vi "ReplaceAngles.vi"(9 "Angle2In":dbl, 10 "Angle1In":dbl, 11 "Comm":T1={"url"="https://rogers.onshape.com/api/partstudios/d/78f5bf641b1754cc5a2885a6/w/2816a0ac3f158e698c5324a2/e/990ec2d1208dce12e8c8d73d/sketches?", "sent headers"="Accept: application/json\r\nAuthorization: On 5WRzTWmAmwc94xTxHfKZAg5i:HmacSHA256:lDyQC1x2JlGNCtdzVGE5L8N41PUpGQIlxBBiesg5jjs=\r\nContent-Type: application/json\r\nDate: Thu, 16 Apr 2020 23:19:12 GMT\r\nOn-Nonce: nlS7Y9rr4jS35A8DK9B3OToU\r\nUser_agent: Onshape Python Sample App", "sent body"="", "headers"="HTTP/1.1 200 OK\r\nServer: nginx\r\nDate: Thu, 16 Apr 2020 23:19:12 GMT\r\nContent-Type: application/json;charset=UTF-8;qs=0.9\r\nContent-Length: 2372\r\nConnection: keep-alive\r\nVary: Accept-Encoding\r\nOn-Version: 1.111.25149.0c1f2eb083aa\r\nOn-Request-Id: a78cc699fde7b461387b36e3\r\nDeprecation: version=UNDEFINED, message=\"You specified mediatype application/json;charset=UTF-8;qs=0.9 and this endpoint will currently accept application/vnd.onshape.v1+json;charset=UTF-8;qs=0.1. Please consider updating to the latest version by specifying application/vnd.onshape.v1+json;charset=UTF-8;qs=0.1 within the Accept header.\r\nSet-Cookie: _u=webservice-3e25a82e; Path=/; Secure; HttpOnly;\r\nX-Frame-Options: SAMEORIGIN\r\nStrict-Transport-Security: max-age=31536000; includeSubDomains\r\nX-Content-Type-Options: nosniff\r\nX-XSS-Protection: 1; mode=block\r\nContent-Security-Policy-Report-Only: object-src 'self' https://embedwistia-a.akamaihd.net; report-uri /api/csp\r\n\r\n", "body"="{\n  \"sketches\" : [ {\n    \"sketch\" : \"Sketch 1\",\n    \"featureId\" : \"FbqM6rYzUBbMRp8_0\",\n    \"transformMatrix\" : [ 1.0, 0.0, 0.0, 0.0, 0.0, 1.0, 0.0, 0.0, 0.0, 0.0, 1.0, 0.0, 0.0, 0.0, 0.0, 1.0 ],\n    \"featuresUsed\" : [ ],\n    \"geomEntities\" : [ {\n      \"id\" : \"C471k0qsEi0Q.start\",\n      \"entityType\" : \"point\",\n      \"point\" : [ 0.017283352091908455, -0.007151731755584478 ]\n    }, {\n      \"id\" : \"C471k0qsEi0Q.end\",\n      \"entityType\" : \"point\",\n      \"point\" : [ -0.04529430344700813, 0.05423396825790405 ]\n    }, {\n      \"id\" : \"C471k0qsEi0Q.0.internal\",\n      \"entityType\" : \"point\",\n      \"point\" : [ 0.017283352091908455, -0.007151731755584478 ]\n    }, {\n      \"id\" : \"C471k0qsEi0Q.1.internal\",\n      \"entityType\" : \"point\",\n      \"point\" : [ 0.05095608904957771, 0.022945139557123184 ]\n    }, {\n      \"id\" : \"C471k0qsEi0Q.2.internal\",\n      \"entityType\" : \"point\",\n      \"point\" : [ 0.02443508431315422, 0.05780983343720436 ]\n    }, {\n      \"id\" : \"C471k0qsEi0Q.3.internal\",\n      \"entityType\" : \"point\",\n      \"point\" : [ -0.018177319318056107, 0.039334528148174286 ]\n    }, {\n      \"id\" : \"C471k0qsEi0Q.4.internal\",\n      \"entityType\" : \"point\",\n      \"point\" : [ -0.04529430344700813, 0.05423396825790405 ]\n    }, {\n      \"id\" : \"C471k0qsEi0Q.startDerivative\",\n      \"entityType\" : \"point\",\n      \"point\" : [ 0.03353424071398461, 8.902966705931049E-4 ],\n      \"isConstruction\" : true\n    }, {\n      \"id\" : \"C471k0qsEi0Q.endDerivative\",\n      \"entityType\" : \"point\",\n      \"point\" : [ -0.0368764138795279, 0.04584760236142172 ],\n      \"isConstruction\" : true\n    }, {\n      \"id\" : \"C471k0qsEi0Q\",\n      \"entityType\" : \"interpolatedSplineSegment\",\n      \"periodic\" : false,\n      \"startHandle\" : [ 0.03353424071398461, 8.902966705931043E-4 ],\n      \"endHandle\" : [ -0.03687641387952791, 0.045847602361421734 ],\n      \"startDerivative\" : [ 0.18655982097041743, 0.0923222980796617 ],\n      \"endDerivative\" : [ -0.1167534466674709, 0.11631622339302505 ],\n      \"interpolationPoints\" : [ [ 0.017283352091908455, -0.007151731755584478 ], [ 0.05095608904957771, 0.022945139557123184 ], [ 0.02443508431315422, 0.05780983343720436 ], [ -0.018177319318056107, 0.039334528148174286 ], [ -0.04529430344700813, 0.05423396825790405 ] ],\n      \"startParameter\" : 0.0,\n      \"endParameter\" : 1.0,\n      \"endPointIds\" : [ \"C471k0qsEi0Q.start\", \"C471k0qsEi0Q.end\" ]\n    } ]\n  } ]\n}", "Sent"="get https://rogers.onshape.com/api/partstudios/d/78f5bf641b1754cc5a2885a6/w/2816a0ac3f158e698c5324a2/e/990ec2d1208dce12e8c8d73d/sketches? \n\nAccept: application/json\r\nAuthorization: On 5WRzTWmAmwc94xTxHfKZAg5i:HmacSHA256:lDyQC1x2JlGNCtdzVGE5L8N41PUpGQIlxBBiesg5jjs=\r\nContent-Type: application/json\r\nDate: Thu, 16 Apr 2020 23:19:12 GMT\r\nOn-Nonce: nlS7Y9rr4jS35A8DK9B3OToU\r\nUser_agent: Onshape Python Sample App\n\n", "Received"="HTTP/1.1 200 OK\r\nServer: nginx\r\nDate: Thu, 16 Apr 2020 23:19:12 GMT\r\nContent-Type: application/json;charset=UTF-8;qs=0.9\r\nContent-Length: 2372\r\nConnection: keep-alive\r\nVary: Accept-Encoding\r\nOn-Version: 1.111.25149.0c1f2eb083aa\r\nOn-Request-Id: a78cc699fde7b461387b36e3\r\nDeprecation: version=UNDEFINED, message=\"You specified mediatype application/json;charset=UTF-8;qs=0.9 and this endpoint will currently accept application/vnd.onshape.v1+json;charset=UTF-8;qs=0.1. Please consider updating to the latest version by specifying application/vnd.onshape.v1+json;charset=UTF-8;qs=0.1 within the Accept header.\r\nSet-Cookie: _u=webservice-3e25a82e; Path=/; Secure; HttpOnly;\r\nX-Frame-Options: SAMEORIGIN\r\nStrict-Transport-Security: max-age=31536000; includeSubDomains\r\nX-Content-Type-Options: nosniff\r\nX-XSS-Protection: 1; mode=block\r\nContent-Security-Policy-Report-Only: object-src 'self' https://embedwistia-a.akamaihd.net; report-uri /api/csp\r\n\r\n\n\n{\n  \"sketches\" : [ {\n    \"sketch\" : \"Sketch 1\",\n    \"featureId\" : \"FbqM6rYzUBbMRp8_0\",\n    \"transformMatrix\" : [ 1.0, 0.0, 0.0, 0.0, 0.0, 1.0, 0.0, 0.0, 0.0, 0.0, 1.0, 0.0, 0.0, 0.0, 0.0, 1.0 ],\n    \"featuresUsed\" : [ ],\n    \"geomEntities\" : [ {\n      \"id\" : \"C471k0qsEi0Q.start\",\n      \"entityType\" : \"point\",\n      \"point\" : [ 0.017283352091908455, -0.007151731755584478 ]\n    }, {\n      \"id\" : \"C471k0qsEi0Q.end\",\n      \"entityType\" : \"point\",\n      \"point\" : [ -0.04529430344700813, 0.05423396825790405 ]\n    }, {\n      \"id\" : \"C471k0qsEi0Q.0.internal\",\n      \"entityType\" : \"point\",\n      \"point\" : [ 0.017283352091908455, -0.007151731755584478 ]\n    }, {\n      \"id\" : \"C471k0qsEi0Q.1.internal\",\n      \"entityType\" : \"point\",\n      \"point\" : [ 0.05095608904957771, 0.022945139557123184 ]\n    }, {\n      \"id\" : \"C471k0qsEi0Q.2.internal\",\n      \"entityType\" : \"point\",\n      \"point\" : [ 0.02443508431315422, 0.05780983343720436 ]\n    }, {\n      \"id\" : \"C471k0qsEi0Q.3.internal\",\n      \"entityType\" : \"point\",\n      \"point\" : [ -0.018177319318056107, 0.039334528148174286 ]\n    }, {\n      \"id\" : \"C471k0qsEi0Q.4.internal\",\n      \"entityType\" : \"point\",\n      \"point\" : [ -0.04529430344700813, 0.05423396825790405 ]\n    }, {\n      \"id\" : \"C471k0qsEi0Q.startDerivative\",\n      \"entityType\" : \"point\",\n      \"point\" : [ 0.03353424071398461, 8.902966705931049E-4 ],\n      \"isConstruction\" : true\n    }, {\n      \"id\" : \"C471k0qsEi0Q.endDerivative\",\n      \"entityType\" : \"point\",\n      \"point\" : [ -0.0368764138795279, 0.04584760236142172 ],\n      \"isConstruction\" : true\n    }, {\n      \"id\" : \"C471k0qsEi0Q\",\n      \"entityType\" : \"interpolatedSplineSegment\",\n      \"periodic\" : false,\n      \"startHandle\" : [ 0.03353424071398461, 8.902966705931043E-4 ],\n      \"endHandle\" : [ -0.03687641387952791, 0.045847602361421734 ],\n      \"startDerivative\" : [ 0.18655982097041743, 0.0923222980796617 ],\n      \"endDerivative\" : [ -0.1167534466674709, 0.11631622339302505 ],\n      \"interpolationPoints\" : [ [ 0.017283352091908455, -0.007151731755584478 ], [ 0.05095608904957771, 0.022945139557123184 ], [ 0.02443508431315422, 0.05780983343720436 ], [ -0.018177319318056107, 0.039334528148174286 ], [ -0.04529430344700813, 0.05423396825790405 ] ],\n      \"startParameter\" : 0.0,\n      \"endParameter\" : 1.0,\n      \"endPointIds\" : [ \"C471k0qsEi0Q.start\", \"C471k0qsEi0Q.end\" ]\n    } ]\n  } ]\n}"}) -> (3 "Payload":string="{\n  \"configurationParameters\" : [ {\n    \"type\" : 1826,\n    \"typeName\" : \"BTMConfigurationParameterQuantity\",\n    \"message\" : {\n      \"quantityType\" : \"ANGLE\",\n      \"rangeAndDefault\" : {\n        \"type\" : 181,\n        \"typeName\" : \"BTQuantityRange\",\n        \"message\" : {\n          \"units\" : \"degree\",\n          \"minValue\": 132.737430,\"maxValue\":132.737430,\"defaultValue\":132.737430,\"location\" : {\n            \"type\" : 226,\n            \"typeName\" : \"BTLocationInfo\",\n            \"message\" : {\n              \"document\" : \"\",\n              \"version\" : \"\",\n              \"topLevel\" : \"\",\n              \"parseNodeId\" : \"\",\n              \"character\" : 0,\n              \"line\" : 0,\n              \"column\" : 0,\n              \"endCharacter\" : 0,\n              \"endLine\" : 0,\n              \"endColumn\" : 0,\n              \"languageVersion\" : 0,\n              \"moduleIds\" : {\n                \"type\" : 1897,\n                \"typeName\" : \"BTDocumentVersionElementIds\",\n                \"message\" : {\n                  \"documentId\" : \"\",\n                  \"versionId\" : \"\",\n                  \"elementId\" : \"\"\n                }\n              },\n              \"elementMicroversion\" : \"\",\n              \"nodeId\" : \"+yByOudIvs1toQrG\"\n            }\n          }\n        }\n      },\n      \"parameterId\" : \"Angle1\",\n      \"parameterName\" : \"Angle1\",\n      \"hasUserCode\" : false,\n      \"nodeId\" : \"MLUebAszJBdGJ1Mml\"\n    }\n  }, {\n    \"type\" : 1826,\n    \"typeName\" : \"BTMConfigurationParameterQuantity\",\n    \"message\" : {\n      \"quantityType\" : \"ANGLE\",\n      \"rangeAndDefault\" : {\n        \"type\" : 181,\n        \"typeName\" : \"BTQuantityRange\",\n        \"message\" : {\n          \"units\" : \"degree\",\n          \"minValue\": 136.759777,\"maxValue\":136.759777,\"defaultValue\":136.759777,\"location\" : {\n            \"type\" : 226,\n            \"typeName\" : \"BTLocationInfo\",\n            \"message\" : {\n              \"document\" : \"\",\n              \"version\" : \"\",\n              \"topLevel\" : \"\",\n              \"parseNodeId\" : \"\",\n              \"character\" : 0,\n              \"line\" : 0,\n              \"column\" : 0,\n              \"endCharacter\" : 0,\n              \"endLine\" : 0,\n              \"endColumn\" : 0,\n              \"languageVersion\" : 0,\n              \"moduleIds\" : {\n                \"type\" : 1897,\n                \"typeName\" : \"BTDocumentVersionElementIds\",\n                \"message\" : {\n                  \"documentId\" : \"\",\n                  \"versionId\" : \"\",\n                  \"elementId\" : \"\"\n                }\n              },\n              \"elementMicroversion\" : \"\",\n              \"nodeId\" : \"nmmgAxmpA3/6A7S2\"\n            }\n          }\n        }\n      },\n      \"parameterId\" : \"Angle2\",\n      \"parameterName\" : \"Angle2\",\n      \"hasUserCode\" : false,\n      \"nodeId\" : \"MNFt8eTIlUIn6Aovo\"\n    }\n  } ],\n  \"currentConfiguration\" : [ ],\n  \"serializationVersion\" : \"1.1.20\",\n  \"sourceMicroversion\" : \"c4ccdcc4397d35da48f1bf8e\",\n  \"rejectMicroversionSkew\" : false,\n  \"microversionSkew\" : false,\n  \"libraryVersion\" : 1458\n}")   [LabVIEW 2020]
uses:
  HTTPComm.ctl
panel:
  in  "error":i32=200
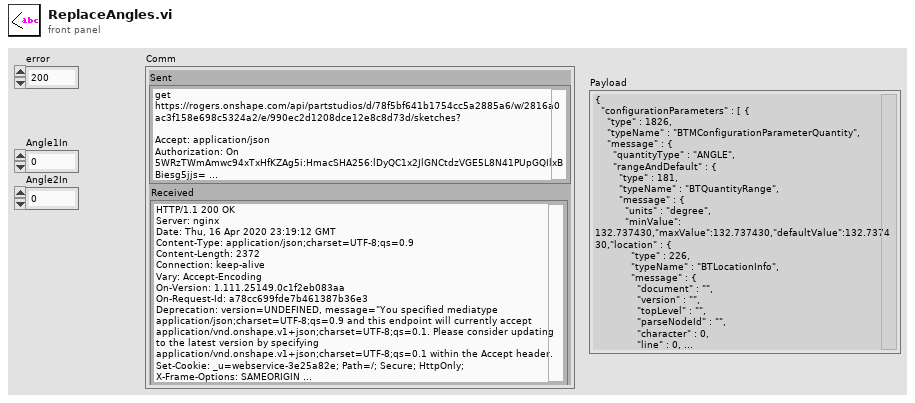
[diagram p1: front panel]
types:
  T1 = typedef "HTTPComm.ctl" = cluster{"url":string, "sent headers":string, "sent body":string, "headers":string, "body":string, "Sent":string, "Received":string}
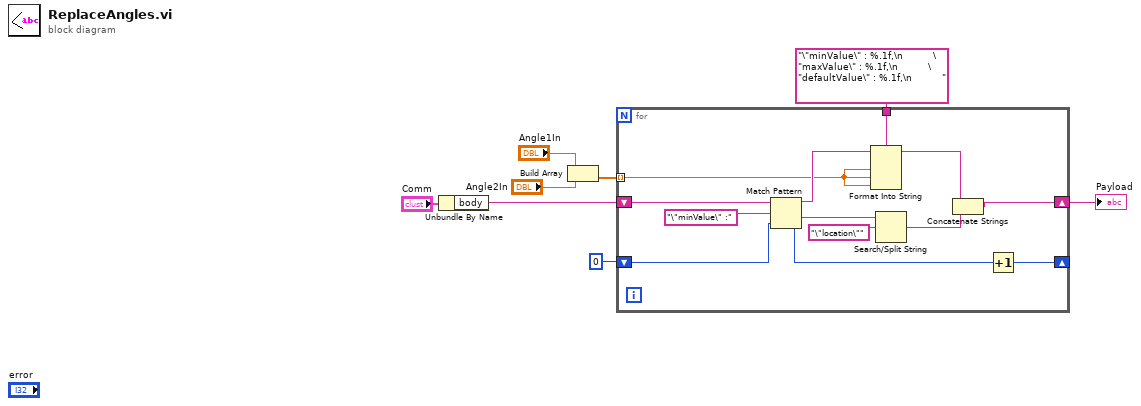
[diagram p0: block diagram]
diagram:
  n1 = Unbundle By Name("Comm") -> ("body"=w5:string)
  n2 = Build Array("Angle1In", "Angle2In") -> (w2:dbl[])
  n3 = for {
    shift-right: [w13] -> w1
    shift-left: w5 -> [w21]
    tunnel: "\"minValue\" : %.1f,\n          \"maxValue\" : %.1f,\n          \"defaultValue\" : %.1f,\n          " ("regular expression") -> [w16]
    shift-right: [w10] -> _
    shift-left: 0 -> [w12]
    tunnel: w2 -> [w9] mode=indexing
    n4 = Match Pattern(string=w21, regular expression="\"minValue\" :", offset (0)=w12) -> (before substring=w17:string, after substring=w19:string, offset past match=w11:i32)  [unwired: 1 out]
    n5 = Format Into String(format string=w16, initial string=w17, w9, w9, w9) -> (resulting string=w15:string)  [unwired: 1 in, 1 out]
    n6 = Search/Split String(string=w19, search string/char (-)="\"location\"" ("regular expression")) -> (match + rest of string=w14:string)  [unwired: 1 in, 2 out]
    n7 = Concatenate Strings(w15, w14) -> (w13:string)
    n8 = Increment(x=w11) -> (x+1=w10:i32)
  }
  "Payload" <- w1
